vi "Close-all-motors.vi"(8 "error in (no error)":errorcluster, 11 "Available motors in":refnum<class "Motor-assembly.lvclass">) -> (0 "error out":errorcluster, 3 "Available motors out":refnum<class "Motor-assembly.lvclass">)   [LabVIEW 2013, in "PowderDeposition.lvlib" / "Motor-assembly.lvclass"]
doc: "Use this template to build a VI to use as a subVI."
uses:
  Motor-assembly.lvclass
  Motor/Motor.lvclass
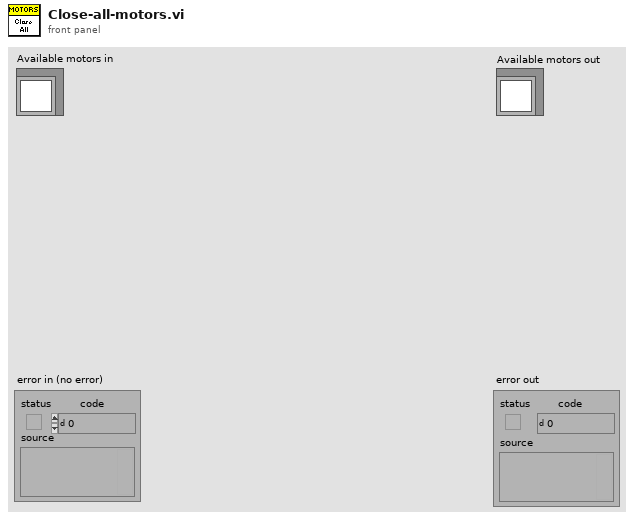
[diagram p1: front panel]
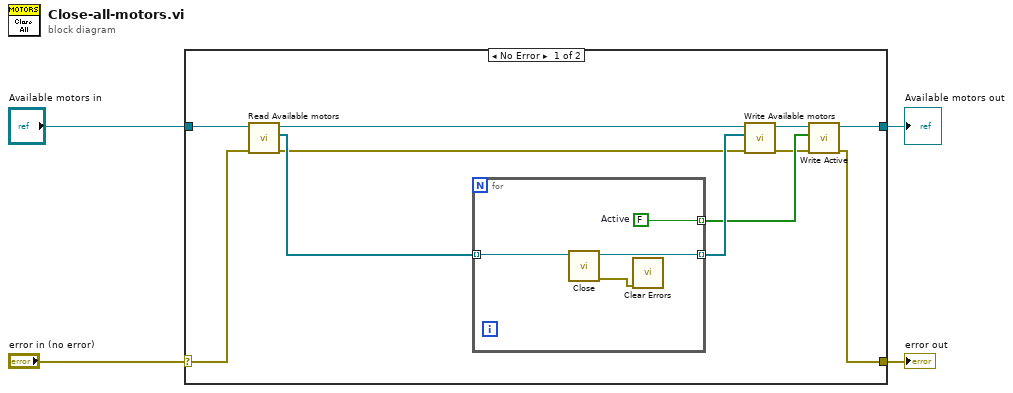
[diagram p0: block diagram]
diagram:
  n1 = case shown="No Error" "error in (no error)" {
    selector: "error in (no error)" -> [w15 w21]
    tunnel: [w9 w21] -> w3
    tunnel: "Available motors in" -> [w8 w20]
    tunnel: [w7 w20] -> w1
    frame No Error {
      n2 = call-dynamic "Read Available motors.vi"("error in (no error)"=w15, "Available motors in"=w8) -> ("error out"=w5:errorcluster, "Available motors"=w14:refnum<class "Motor.lvclass">[], "Available motors out"=w6:refnum<class "Motor-assembly.lvclass">)  [unwired: 7 in]
      n3 = for {
        tunnel: w14 -> [w19] mode=indexing
        tunnel: [w18] -> w13 mode=indexing
        tunnel: [w17] -> w12 mode=indexing
        w17 = FALSE  # Active
        n4 = call-dynamic "Close.vi"("Motor in"=w19) -> ("error out"=w16:errorcluster, "Motor out"=w18:refnum<class "Motor.lvclass">)  [unwired: 9 in]
        n5 = call <vilib>:"Clear Errors.vi"("error in (no error)"=w16) -> ()  [unwired: 6 in, 1 out]
      }
      n6 = call-dynamic "Write Available motors.vi"("error in (no error)"=w5, "Available motors"=w13, "Available motors in"=w6) -> ("error out"=w10:errorcluster, "Available motors out"=w11:refnum<class "Motor-assembly.lvclass">)  [unwired: 7 in]
      n7 = call-dynamic "Write Active.vi"("error in (no error)"=w10, "Active?"=w12, "Available motors in"=w11) -> ("error out"=w9:errorcluster, "Available motors out"=w7:refnum<class "Motor-assembly.lvclass">)  [unwired: 7 in]
    }
    frame Error {
    }
  }
  "error out" <- w3
  "Available motors out" <- w1
